vi "Wolna nadawanie nazw.vi"(8 "error in (no error)":errorcluster, 11 "Rejestracja in":T1) -> (0 "error out":errorcluster, 3 "Rejestracja out":T1)   [LabVIEW 2014]
doc: "Nadaje opisy przebiegom w akwizycji wolnej\nna podstawie typu rejestracji i numerów kanału"
uses:
  Kontrolki/GUI/RejWol_konfig_opis GUI.ctl
  Kontrolki/GUI/RejWol_typ.ctl
  Kontrolki/GUI/RejWol_numer_kanalu.ctl
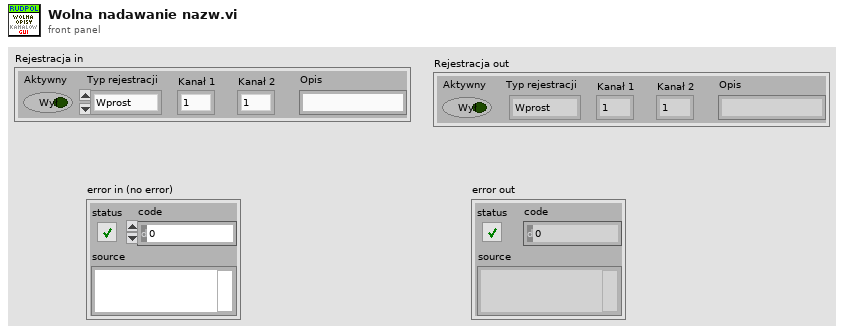
[diagram p1: front panel]
types:
  T1 = typedef "RejWol_konfig_opis GUI.ctl" = cluster{"Typ rejestracji":T2, "Opis":string, "Aktywny":bool, "Kanał 1":T3, "Kanał 2":T3}
  T2 = typedef "RejWol_typ.ctl" = enum16{"Wprost", "Moduł", "Kwadrat", "Iloczyn", "Faza"}
  T3 = typedef "RejWol_numer_kanalu.ctl" = enum16{"1", "2", "3", "4", "5", "6", "7", "8"}
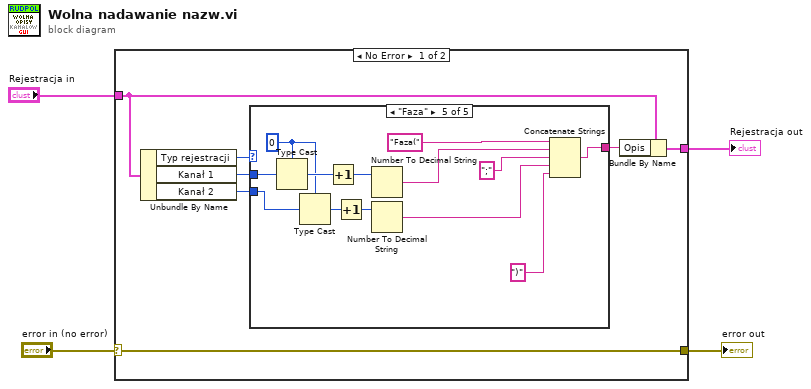
[diagram p0: block diagram]
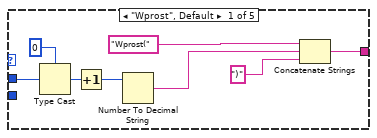
[diagram p2: hidden frame]
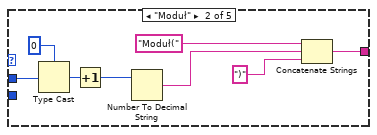
[diagram p3: hidden frame]
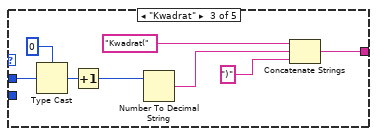
[diagram p4: hidden frame]
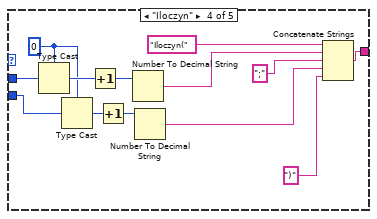
[diagram p5: hidden frame]
diagram:
  n1 = case shown="No Error" "error in (no error)" {
    selector: "error in (no error)" -> [w7 w62]
    tunnel: [w11 w63] -> w1
    tunnel: "Rejestracja in" -> [w9 w63]
    tunnel: [w7 w62] -> w3
    frame No Error {
      n2 = Unbundle By Name(w9) -> ("Typ rejestracji"=w8:T2, "Kanał 1"=w6:T3, "Kanał 2"=w5:T3)
      n3 = case shown="\"Faza\"" w8 {
        tunnel: w6 -> [w15 w21 w29 w41 w52]
        tunnel: [w16 w25 w33 w48 w57] -> w10
        tunnel: w5 -> [_ _ _ w39 w51]
        frame "Wprost", Default {
          n4 = Type Cast(type=u16 0, x=w15) -> (*(type *) &x=w13:u16)
          n5 = Increment(x=w13) -> (x+1=w12:u16)
          n6 = Number To Decimal String(number=w12) -> (decimal integer string=w19:string)  [unwired: 1 in]
          n7 = Concatenate Strings("Wprost(", w19, ")") -> (w16:string)
        }
        frame "Moduł" {
          n8 = Type Cast(type=u16 0, x=w21) -> (*(type *) &x=w22:u16)
          n9 = Increment(x=w22) -> (x+1=w20:u16)
          n10 = Number To Decimal String(number=w20) -> (decimal integer string=w27:string)  [unwired: 1 in]
          n11 = Concatenate Strings("Moduł(", w27, ")") -> (w25:string)
        }
        frame "Kwadrat" {
          n12 = Type Cast(type=u16 0, x=w29) -> (*(type *) &x=w30:u16)
          n13 = Increment(x=w30) -> (x+1=w28:u16)
          n14 = Number To Decimal String(number=w28) -> (decimal integer string=w35:string)  [unwired: 1 in]
          n15 = Concatenate Strings("Kwadrat(", w35, ")") -> (w33:string)
        }
        frame "Iloczyn" {
          w36 = u16 0
          n16 = Type Cast(type=w36, x=w41) -> (*(type *) &x=w42:u16)
          n17 = Type Cast(type=w36, x=w39) -> (*(type *) &x=w38:u16)
          n18 = Increment(x=w42) -> (x+1=w40:u16)
          n19 = Increment(x=w38) -> (x+1=w37:u16)
          n20 = Number To Decimal String(number=w40) -> (decimal integer string=w46:string)  [unwired: 1 in]
          n21 = Number To Decimal String(number=w37) -> (decimal integer string=w45:string)  [unwired: 1 in]
          n22 = Concatenate Strings("Iloczyn(", w46, ";", w45, ")") -> (w48:string)
        }
        frame "Faza" {
          w53 = u16 0
          n23 = Type Cast(type=w53, x=w52) -> (*(type *) &x=w55:u16)
          n24 = Type Cast(type=w53, x=w51) -> (*(type *) &x=w54:u16)
          n25 = Increment(x=w55) -> (x+1=w49:u16)
          n26 = Increment(x=w54) -> (x+1=w50:u16)
          n27 = Number To Decimal String(number=w49) -> (decimal integer string=w61:string)  [unwired: 1 in]
          n28 = Number To Decimal String(number=w50) -> (decimal integer string=w60:string)  [unwired: 1 in]
          n29 = Concatenate Strings("Faza(", w61, ";", w60, ")") -> (w57:string)
        }
      }
      n30 = Bundle By Name(cluster=w9, "Opis"=w10) -> (w11:T1)
    }
    frame Error {
    }
  }
  "error out" <- w3
  "Rejestracja out" <- w1
